vi "REFAIRE.vi"(1 "image":string, 4 "use Jerome?":bool=TRUE, 5 "CAS REFAIRE":T1=enum."Crash", 6 "Pédale":bool, 7 "CAS OK":T1=enum."Crash", 8 "errin":errorcluster, 9 "test ok ?":bool, 10 "MSG Jerome":string, 11 "Visa Pedale":refnum<visa-resource-name>) -> (0 "errout":errorcluster, 3 "nextstep":T1)   [LabVIEW 2020]
uses:
  10-ZEN35-PkOp/SubVi/state.ctl
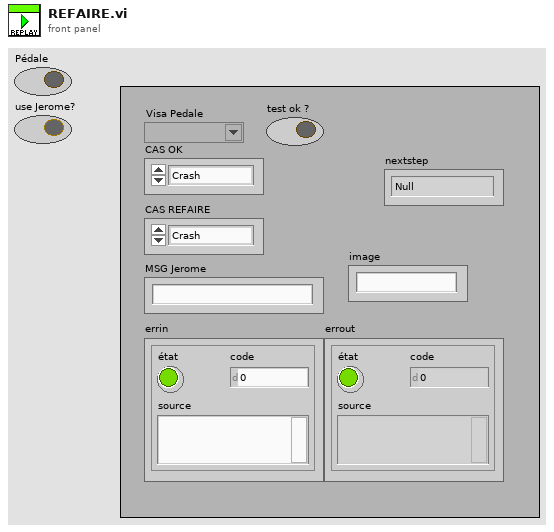
[diagram p1: front panel]
types:
  T1 = typedef "state.ctl" = enum16{"Null", "Demarrage", "Montage", "Verification PV existant", "arrêt", "Bilan OF", "etiquettes inviola", "fin", "rangement diag report", "Déconnection du pack", "impressions", "Cache connecteur J1", "Impression étiquette", "Crash", "report valeurs", "Continuite", "ISO", "Soft PDU CMOD", "Adressage", "SOFT BMS", "DTC", "Test a vide", "diag report", "off", "Scan", "Init"}
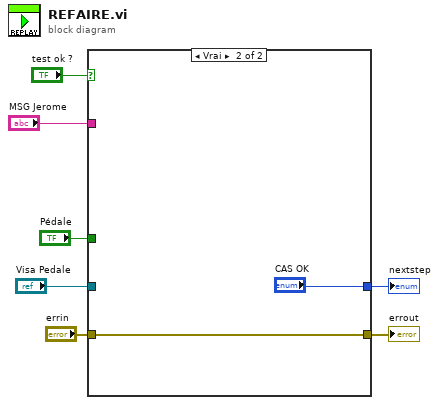
[diagram p0: block diagram]
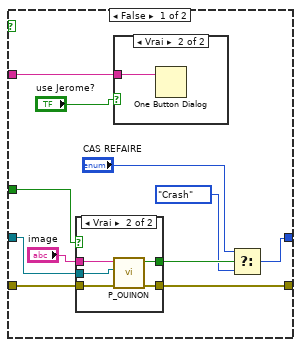
[diagram p2: hidden frame]
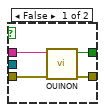
[diagram p4: hidden frame]
diagram:
  n1 = case shown="Vrai" "test ok ?" {
    tunnel: "errin" -> [w18 w30]
    tunnel: [w17 w30] -> w6
    tunnel: "Visa Pedale" -> [w15 _]
    tunnel: [w13 "CAS OK"] -> w7
    tunnel: "MSG Jerome" -> [w12 _]
    tunnel: "Pédale" -> [w11 _]
    frame False {
      n2 = case shown="Vrai" w11 {
        tunnel: "image" -> [w20 w28]
        tunnel: w18 -> [w23 w27]
        tunnel: [w22 w26] -> w17
        tunnel: [w21 w25] -> w16
        tunnel: w15 -> [_ w24]
        frame False {
          n3 = call <userlib>:"OUINON.vi"("errin"=w23, "image"=w20) -> ("error out"=w22:errorcluster, "Booléen"=w21:bool)  [unwired: 8 in]
        }
        frame True {
          n4 = call <userlib>:"P_OUINON.vi"("errin"=w27, "VISAin"=w24, "Image"=w28) -> ("error out"=w26:errorcluster, "=OUI?"=w25:bool)  [unwired: 7 in]
        }
      }
      n5 = case shown="Vrai" "use Jerome?" {
        tunnel: w12 -> [_ w19]
        frame False {
        }
        frame True {
          n6 = One Button Dialog(message=w19) -> ()  [unwired: 1 in, 1 out]
        }
      }
      n7 = Select(t="CAS REFAIRE", s=w16, f=state."Crash") -> (s? t:f=w13:T1)
    }
    frame True {
    }
  }
  "nextstep" <- w7
  "errout" <- w6
